vi "Bounding Box to Corner Points.vi"(1 "Bounding Box":T2) -> (0 "Rectangle Points Out":T1)   [LabVIEW 2011]
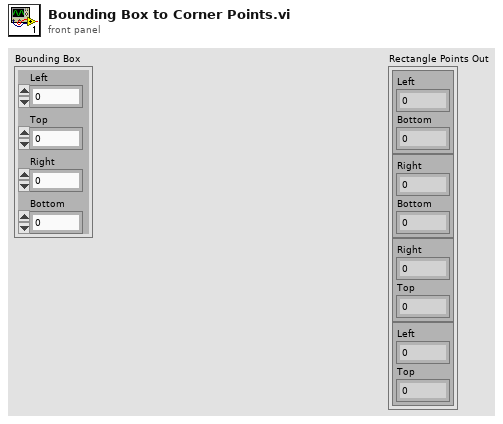
[diagram p1: front panel]
types:
  T1 = cluster{cluster{"Left":dbl, "Bottom":dbl}, cluster{"Right":dbl, "Bottom":dbl}, cluster{"Right":dbl, "Top":dbl}, cluster{"Left":dbl, "Top":dbl}}
  T2 = cluster{"Left":dbl, "Top":dbl, "Right":dbl, "Bottom":dbl}
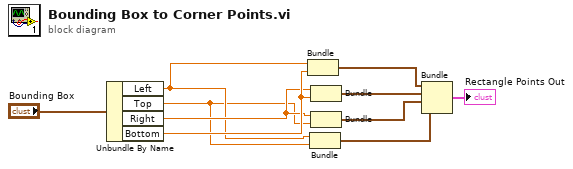
[diagram p0: block diagram]
diagram:
  n1 = Unbundle By Name("Bounding Box") -> ("Left"=w7:dbl, "Top"=w6:dbl, "Right"=w8:dbl, "Bottom"=w9:dbl)
  n2 = Bundle("Left"=w7, "Bottom"=w9) -> (w5:cluster{"Left":dbl, "Bottom":dbl})  [unwired: 1 in]
  n3 = Bundle("Left"=w7, "Top"=w6) -> (w2:cluster{"Left":dbl, "Top":dbl})  [unwired: 1 in]
  n4 = Bundle("Right"=w8, "Bottom"=w9) -> (w4:cluster{"Right":dbl, "Bottom":dbl})  [unwired: 1 in]
  n5 = Bundle("Right"=w8, "Top"=w6) -> (w3:cluster{"Right":dbl, "Top":dbl})  [unwired: 1 in]
  n6 = Bundle(w5, w4, w3, w2) -> (→"Rectangle Points Out":T1)  [unwired: 1 in]
